vi "Frame Counter.vi"(6 "init? (F)":bool, 7 "bus type":enum16{"CAN", "FlexRay", "LIN"}(ring), 8 "error in (no error)":errorcluster, 9 "new frames":i32, 11 "bus index (bus count for init)":i32) -> (0 "error out":errorcluster, 1 "total frames":u32)   [LabVIEW 2018, in "NI-XNET Monitor Engine.lvlib"]
uses:
  NI-XNET Monitor Engine.lvlib
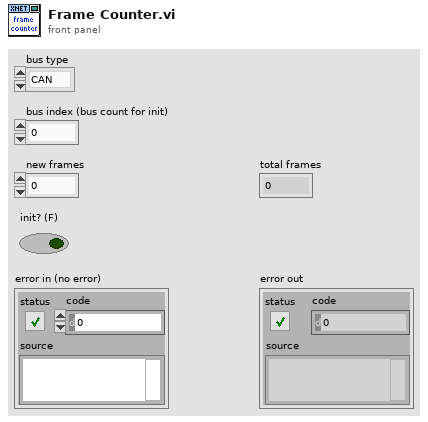
[diagram p1: front panel]
types:
  T1 = cluster{"CAN":u32[], "FlexRay":u32[], "LIN":u32[]}
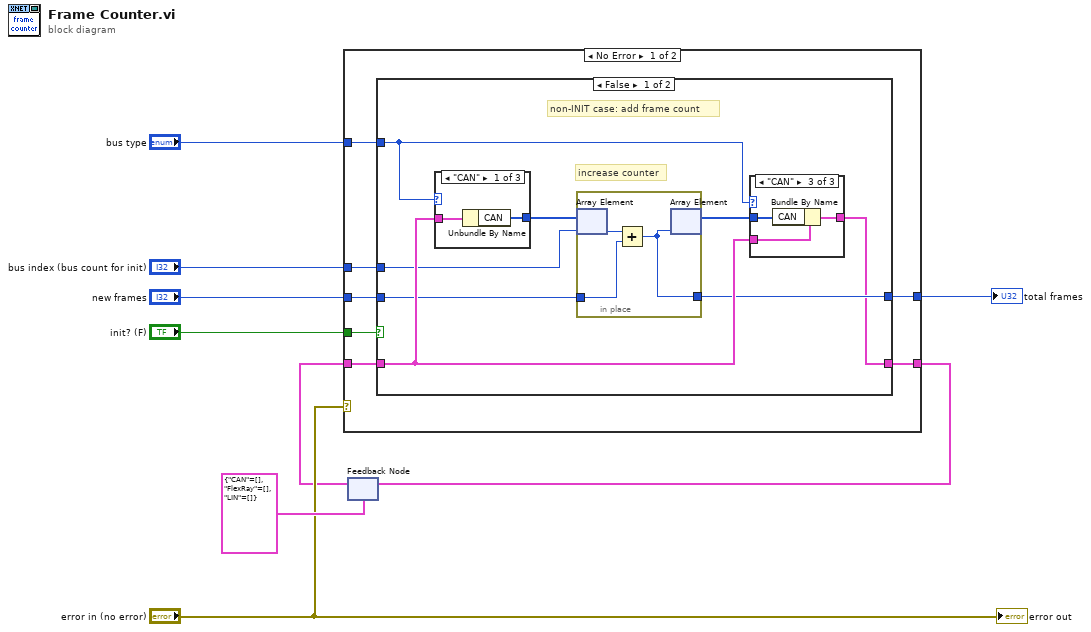
[diagram p0: block diagram]
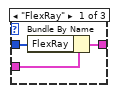
[diagram p2: hidden frame]
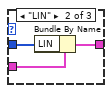
[diagram p3: hidden frame]
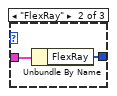
[diagram p4: hidden frame]
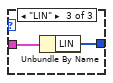
[diagram p5: hidden frame]
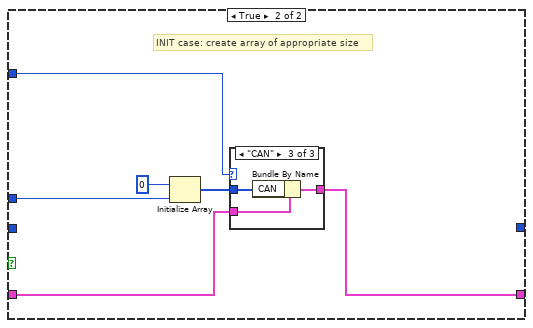
[diagram p6: hidden frame]
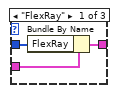
[diagram p7: hidden frame]
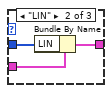
[diagram p8: hidden frame]
diagram:
  n1 = feedback #1(T1 {"CAN"=[], "FlexRay"=[], "LIN"=[]} ("Frames counter")) -> (w1:T1)
  n2 = case shown="No Error" "error in (no error)" {
    tunnel: "bus type" -> [w16 _]
    tunnel: w1 -> [w15 w58]
    tunnel: "bus index (bus count for init)" -> [w14 _]
    tunnel: "new frames" -> [w13 _]
    tunnel: [w12 _] -> w5
    tunnel: [w11 w58] -> w4
    tunnel: "init? (F)" -> [w10 _]
    frame No Error {
      n3 = case shown="False" w10 {
        tunnel: w16 -> [w24 w48]
        tunnel: w15 -> [w23 w47]
        tunnel: w14 -> [w20 w45]
        tunnel: w13 -> [w19 _]
        tunnel: [w18 _] -> w12
        tunnel: [w17 w46] -> w11
        frame False {
          # "non-INIT case: add frame count"
          # "increase counter"
          n4 = case shown="\"CAN\"" w24 {
            tunnel: w23 -> [w38 w40 w42]
            tunnel: [w37 w39 w41] -> w21
            frame "CAN" {
              n5 = Unbundle By Name(w38) -> ("CAN"=w37:u32[])
            }
            frame "FlexRay" {
              n6 = Unbundle By Name(w40) -> ("FlexRay"=w39:u32[])
            }
            frame "LIN" {
              n7 = Unbundle By Name(w42) -> ("LIN"=w41:u32[])
            }
          }
          n8 = in-place {
            in-place-border: w19 -> [w26]
            in-place-border: [w25] -> w18
            n9 = in-place-array #2(w21, w20) -> (w27:u32)
            n10 = Add(x=w27, y=w26) -> (x+y=w25:u32)
            n11 = in-place-array #2(w25) -> (w22:u32[])  [unwired: 1 out]
          }
          n12 = case shown="\"CAN\"" w24 {
            tunnel: w23 -> [w29 w32 w35]
            tunnel: w22 -> [w30 w33 w36]
            tunnel: [w28 w31 w34] -> w17
            frame "FlexRay" {
              n13 = Bundle By Name(cluster=w29, "FlexRay"=w30) -> (w28:T1)
            }
            frame "LIN" {
              n14 = Bundle By Name(cluster=w32, "LIN"=w33) -> (w31:T1)
            }
            frame "CAN" {
              n15 = Bundle By Name(cluster=w35, "CAN"=w36) -> (w34:T1)
            }
          }
        }
        frame True {
          # "INIT case: create array of appropriate size"
          n16 = Initialize Array(u32 0, w45) -> (w43:u32[])
          n17 = case shown="\"CAN\"" w48 {
            tunnel: w47 -> [w50 w53 w56]
            tunnel: w43 -> [w51 w54 w57]
            tunnel: [w49 w52 w55] -> w46
            frame "FlexRay" {
              n18 = Bundle By Name(cluster=w50, "FlexRay"=w51) -> (w49:T1)
            }
            frame "LIN" {
              n19 = Bundle By Name(cluster=w53, "LIN"=w54) -> (w52:T1)
            }
            frame "CAN" {
              n20 = Bundle By Name(cluster=w56, "CAN"=w57) -> (w55:T1)
            }
          }
        }
      }
    }
    frame Error {
    }
  }
  "total frames" <- w5
  n21 = feedback-in #1(w4) -> ()
  "error out" <- "error in (no error)"
